vi "main.vi"() -> ()   [LabVIEW 2018]
uses:
  <vilib>/Instr/_visa.llb/VISA Configure Serial Port (Instr).vi
panel:
  in  "Velocità":i32(slide) scale=5.0..255.0
  out "Distanza (cm)":dbl
  out "Comando Automatico":string
  out "Velocità":string
  out "Comando Manuale":string
  out "Misura Sensore Distanza":dbl(graph)
  in  "Soglia":cluster{dbl, dbl}(slide)={0.0, 2.3061224489795915} scale=0.05..300.0
  out "Gauge":i32(knob) scale=5.0..255.0
  out "Modalità manuale":bool
  in  "stop":bool
  in  "Guida\nAutomatica /Manuale":bool
  in  "Stop":bool
  in  "Destra":bool
  in  "Sinistra":bool
  in  "Avanti":bool
  in  "Indietro":bool
  out "Status":bool
  in  "VISA resource name":refnum<visa-resource-name>
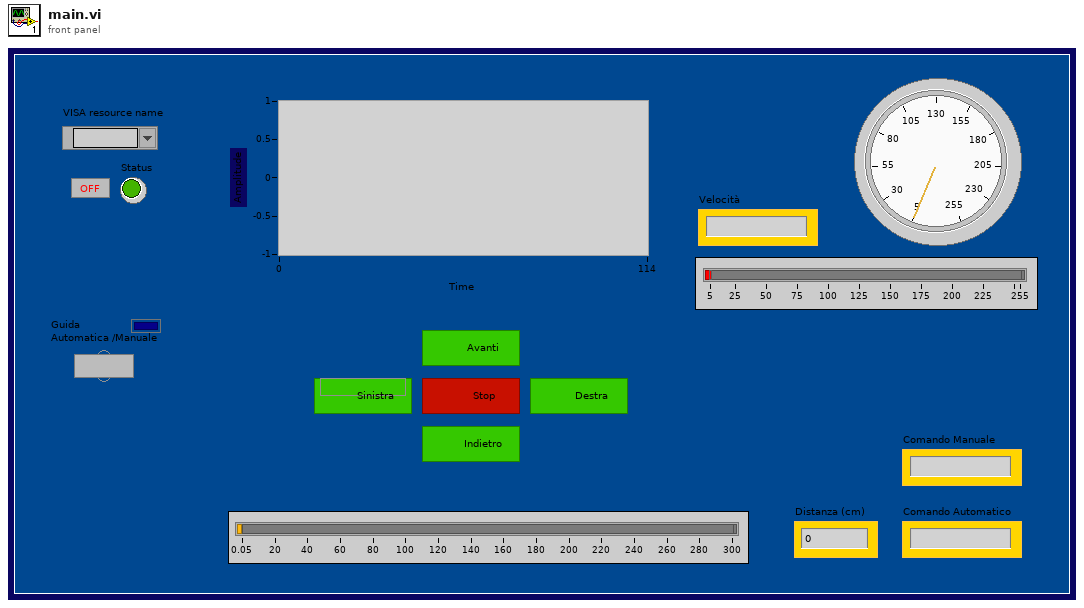
[diagram p1: front panel]
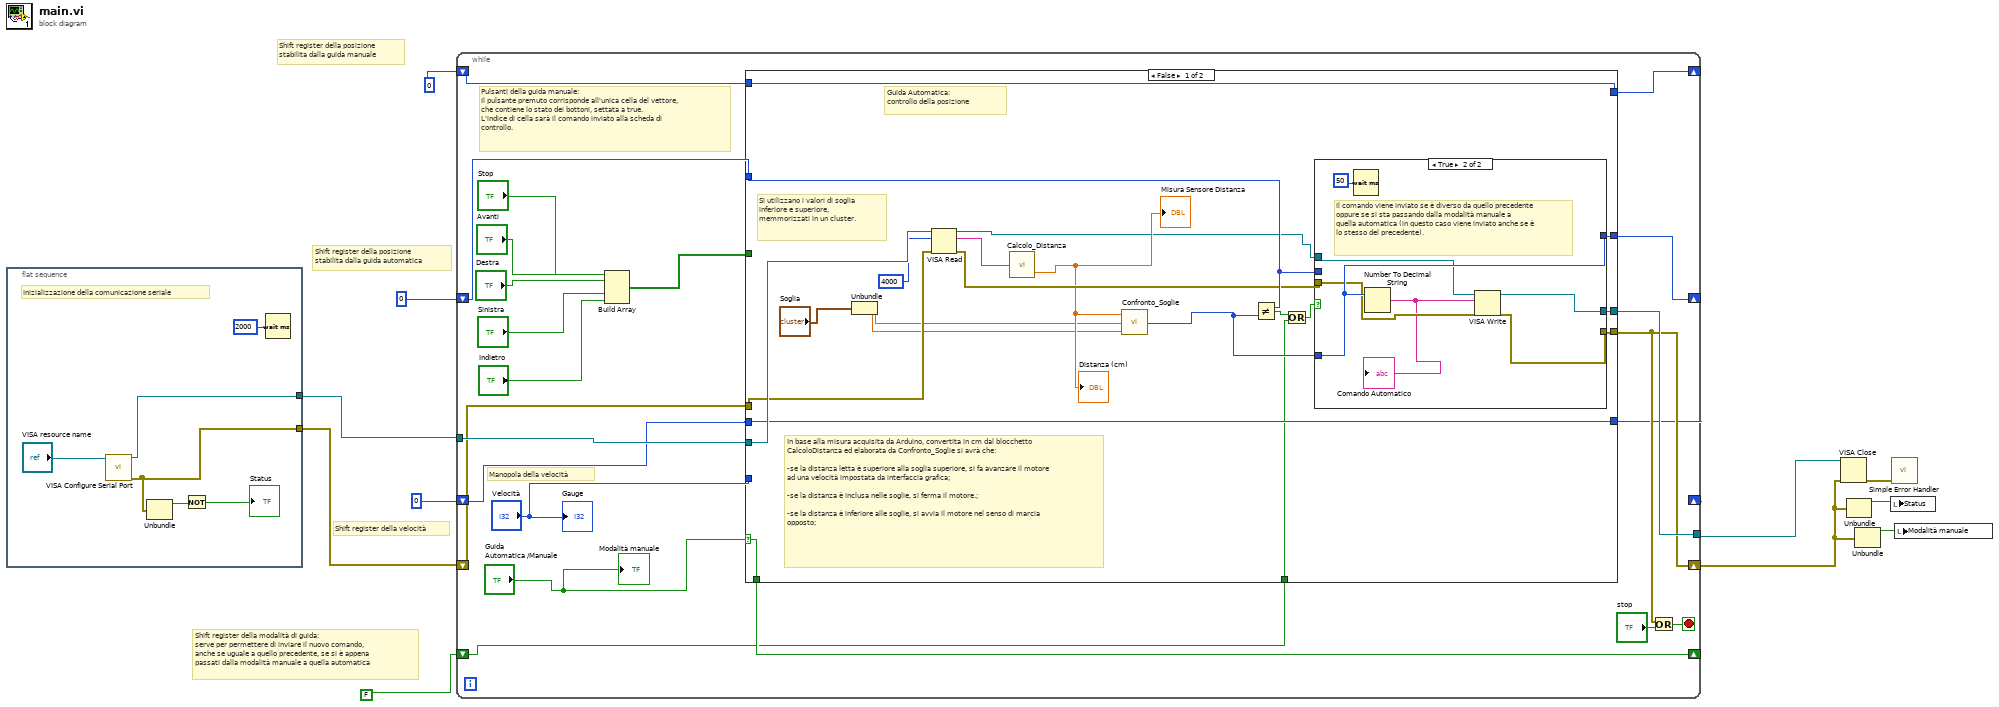
[diagram p0: block diagram]
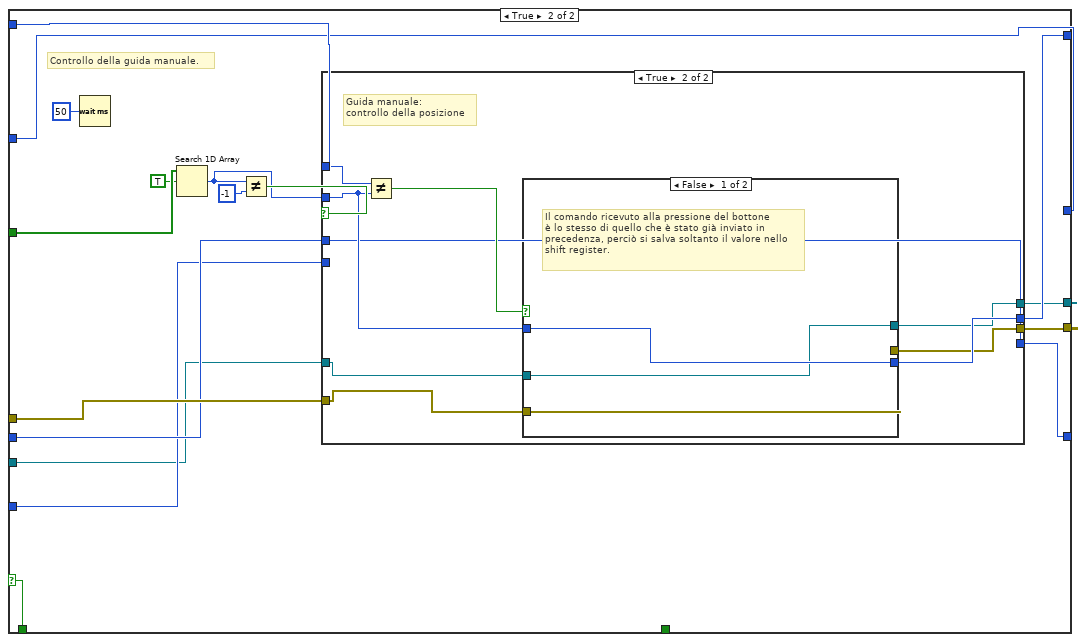
[diagram p3: hidden frame]
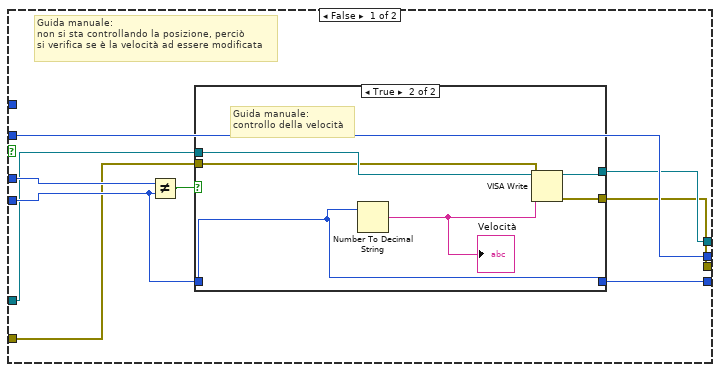
[diagram p4: hidden frame]
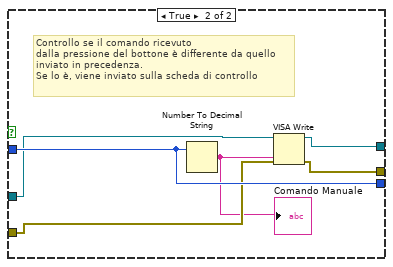
[diagram p6: hidden frame]
diagram:
  # "Shift register della modalità di guida:\nserve per permettere di inviare il nuovo comando,\nanche se uguale a quello precedente, se si è appena\npassati dalla modalità manuale a quella automatica"
  # "Shift register della posizione \nstabilita dalla guida automatica"
  # "Shift register della velocità"
  # "Shift register della posizione\nstabilita dalla guida manuale"
  n1 = flat-sequence {
    tunnel: [w16] -> w7
    tunnel: [w15] -> w6
    frame #0 {
      # "Inizializzazione della comunicazione seriale"
      n2 = call-poly "VISA Configure Serial Port"("VISA resource name"="VISA resource name") -> ("VISA resource name out"=w16:refnum<visa-resource-name>, "error out"=w15:errorcluster)  [unwired: 13 in]
      n3 = Unbundle(w15) -> ("status"=w14:bool)  [unwired: 2 out]
      n4 = Not(x=w14) -> (.not. x?=→"Status":bool)
      n5 = Wait (ms)(milliseconds to wait=u32 2000) -> ()  [unwired: 1 out]
    }
  }
  n6 = while {
    shift-right: [w31] -> _
    shift-left: 0 -> [w32]
    shift-right: [w21] -> _
    shift-left: 0 -> [w22]
    shift-right: [w28] -> _
    shift-left: 0 -> [w27]
    tunnel: w7 -> [w26]
    shift-right: [w23] -> w3
    shift-left: w6 -> [w25]
    tunnel: [w24] -> w5
    shift-right: [w19] -> _
    shift-left: FALSE -> [w18]
    stop <- w39 stop-if-true
    # "Manopola della velocità"
    # "Pulsanti della guida manuale:\nIl pulsante premuto corrisponde all'unica cella del vettore, che contiene lo stato dei bottoni, settata a true.\nL'indice di cella sarà il comando inviato alla scheda di controllo."
    n7 = Build Array("Stop", "Avanti", "Destra", "Sinistra", "Indietro") -> (w38:bool[])
    n8 = case shown="False" "Guida\nAutomatica /Manuale" {
      selector: "Guida\nAutomatica /Manuale" -> [w44 w71]
      tunnel: w38 -> [_ w87]
      tunnel: w32 -> [w51 w82]
      tunnel: [w51 w81] -> w31
      tunnel: [w57 w80] -> w28
      tunnel: w27 -> [w58 w80]
      tunnel: w26 -> [w56 w74]
      tunnel: w25 -> [w55 w79]
      tunnel: [w52 w78] -> w23
      tunnel: [w53 w77] -> w24
      tunnel: w22 -> [w50 w76]
      tunnel: "Velocità" -> [_ w75]
      tunnel: [w50 w72] -> w21
      tunnel: [w44 w71] -> w19
      tunnel: w18 -> [w40 _]
      frame False {
        # "Si utilizzano i valori di soglia inferiore e superiore, memmorizzati in un cluster."
        # "In base alla misura acquisita da Arduino, convertita in cm dal blocchetto CalcoloDistanza ed elaborata da Confronto_Soglie si avrà che:\n\n-se la distanza letta è superiore alla soglia superiore, si fa avanzare il motore ad una velocità impostata da interfaccia grafica;\n\n-se la distanza è inclusa nelle soglie, si ferma il motore.;\n\n-se la distanza è inferiore alle soglie, si avvia il motore nel senso di marcia opposto;"
        # "Guida Automatica:\ncontrollo della posizione"
        n9 = Unbundle("Soglia") -> (w46:dbl, w45:dbl)
        n10 = VISA Read(VISA resource name=w56, byte count=u32 4000, error in (no error)=w55) -> (VISA resource name out=w43:refnum<visa-resource-name>, read buffer=w60:string, error out=w54:errorcluster)  [unwired: 1 out]
        n11 = call "Calcolo_Distanza.vi"("Ingresso in MicroSecondi"=w60) -> ("Centimetri"=w48:dbl)  [unwired: 1 out]
        "Misura Sensore Distanza" <- w48
        "Distanza (cm)" <- w48
        n12 = call "Confronto_Soglie.vi"("max"=w45, "min"=w46, "distanza"=w48) -> ("Comando"=w59:i32)
        n13 = Not Equal?(x=w58, y=w59) -> (x != y?=w42:bool)
        n14 = Or(x=w42, y=w40) -> (x .or. y?=w41:bool)
        n15 = case shown="True" w41 {
          tunnel: w59 -> [_ w69]
          tunnel: [w63 w69] -> w57
          tunnel: w58 -> [w63 _]
          tunnel: w43 -> [w62 w68]
          tunnel: w54 -> [w61 w67]
          tunnel: [w62 w66] -> w53
          tunnel: [w61 w65] -> w52
          frame False {
            # "Se il comando elaborato dalla guida automatica è lo stesso di quello inviato in precedenza si mantiene soltanto il suo valore nello shift register."
          }
          frame True {
            # "Il comando viene inviato se è diverso da quello precedente oppure se si sta passando dalla modalità manuale a quella automatica (in questo caso viene inviato anche se è lo stesso del precedente)."
            n16 = Wait (ms)(milliseconds to wait=u32 50) -> ()  [unwired: 1 out]
            n17 = Number To Decimal String(number=w69) -> (decimal integer string=w64:string)  [unwired: 1 in]
            "Comando Automatico" <- w64
            n18 = VISA Write(VISA resource name=w68, write buffer=w64, error in (no error)=w67) -> (VISA resource name out=w66:refnum<visa-resource-name>, error out=w65:errorcluster)  [unwired: 1 out]
          }
        }
      }
      frame True {
        # "Controllo della guida manuale."
        n19 = Wait (ms)(milliseconds to wait=u32 50) -> ()  [unwired: 1 out]
        n20 = Search 1D Array(1D array=w87, element=TRUE) -> (index of element=w83:i32)  [unwired: 1 in]
        n21 = Not Equal?(x=w83, y=-1) -> (x != y?=w84:bool)
        n22 = case shown="True" w84 {
          tunnel: w83 -> [w96 w112]
          tunnel: w82 -> [_ w114]
          tunnel: [w96 w111] -> w81
          tunnel: w74 -> [w92 w110]
          tunnel: w79 -> [w91 w109]
          tunnel: [w88 w107] -> w78
          tunnel: [w89 w108] -> w77
          tunnel: w76 -> [w94 w106]
          tunnel: w75 -> [w93 _]
          tunnel: [w90 w106] -> w72
          frame False {
            # "Guida manuale:\nnon si sta controllando la posizione, perciò\nsi verifica se è la velocità ad essere modificata"
            n23 = Not Equal?(x=w94, y=w93) -> (x != y?=w95:bool)
            n24 = case shown="True" w95 {
              tunnel: w92 -> [w99 w105]
              tunnel: w91 -> [w98 w104]
              tunnel: [w99 w103] -> w89
              tunnel: [w98 w102] -> w88
              tunnel: [w97 w101] -> w90
              tunnel: w93 -> [w97 w101]
              frame False {
                # "Il valore ricevuto della velocità è lo stesso di quello che è stato già inviato in\nprecedenza, perciò si salva soltanto il valore nello shift register."
              }
              frame True {
                # "Guida manuale:\ncontrollo della velocità"
                n25 = Number To Decimal String(number=w101) -> (decimal integer string=w100:string)  [unwired: 1 in]
                "Velocità" <- w100
                n26 = VISA Write(VISA resource name=w105, write buffer=w100, error in (no error)=w104) -> (VISA resource name out=w103:refnum<visa-resource-name>, error out=w102:errorcluster)  [unwired: 1 out]
              }
            }
          }
          frame True {
            # "Guida manuale:\ncontrollo della posizione"
            n27 = Not Equal?(x=w114, y=w112) -> (x != y?=w113:bool)
            n28 = case shown="False" w113 {
              tunnel: w112 -> [w117 w123]
              tunnel: [w117 w123] -> w111
              tunnel: w110 -> [w116 w122]
              tunnel: w109 -> [w115 w121]
              tunnel: [w116 w120] -> w108
              tunnel: [w115 w119] -> w107
              frame False {
                # "Il comando ricevuto alla pressione del bottone\nè lo stesso di quello che è stato già inviato in\nprecedenza, perciò si salva soltanto il valore nello\nshift register."
              }
              frame True {
                # "Controllo se il comando ricevuto\ndalla pressione del bottone è differente da quello\ninviato in precedenza.\nSe lo è, viene inviato sulla scheda di controllo"
                n29 = Number To Decimal String(number=w123) -> (decimal integer string=w118:string)  [unwired: 1 in]
                "Comando Manuale" <- w118
                n30 = VISA Write(VISA resource name=w122, write buffer=w118, error in (no error)=w121) -> (VISA resource name out=w120:refnum<visa-resource-name>, error out=w119:errorcluster)  [unwired: 1 out]
              }
            }
          }
        }
      }
    }
    n31 = Or(x=w23, y="stop") -> (x .or. y?=w39:bool)
    "Modalità manuale" <- "Guida\nAutomatica /Manuale"
    "Gauge" <- "Velocità"
  }
  n32 = VISA Close(VISA resource name=w5, error in (no error)=w3) -> (error out=w4:errorcluster)
  n33 = Unbundle(w3) -> ("status"=w10:bool)  [unwired: 2 out]
  n34 = Unbundle(w3) -> ("status"=w2:bool)  [unwired: 2 out]
  n35 = local write "Status"(w10) -> ()
  n36 = call <vilib>:"Simple Error Handler.vi"("error in (no error)"=w4) -> ()  [unwired: 4 in, 5 out]
  n37 = local write "Modalità manuale"(w2) -> ()
